vi "Connect.vi"(8 "error in":errorcluster, 11 "ThorlabsLabJack in":refnum<class "ThorlabsLabJack.lvclass">) -> (0 "error out":errorcluster, 3 "ThorlabsLabJack out":refnum<class "ThorlabsLabJack.lvclass">)   [LabVIEW 2018, in "ThorlabsLabJack.lvlib" / "ThorlabsLabJack.lvclass"]
uses:
  ThorlabsLabJack.lvclass
  ThorlabsLabJack.lvclass/ThorlabsLabJack.ctl
  C:/AME Test Engineering/LabVIEW/PPLs/Axis/Thorlabs/Thorlabs.MotionControl.IntegratedStepperMotorsCLI.dll
  PPLs/Axis/Thorlabs/Thorlabs.MotionControl.IntegratedStepperMotorsCLI.dll
  PPLs/Axis/Parent/Axis.lvlibp/Axis.lvclass
  C:/Projects/LWS_Base/trunk/LabVIEW/PPLs/Configuration/Axis.lvlibp/Axis.lvclass
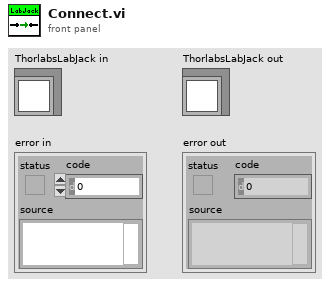
[diagram p1: front panel]
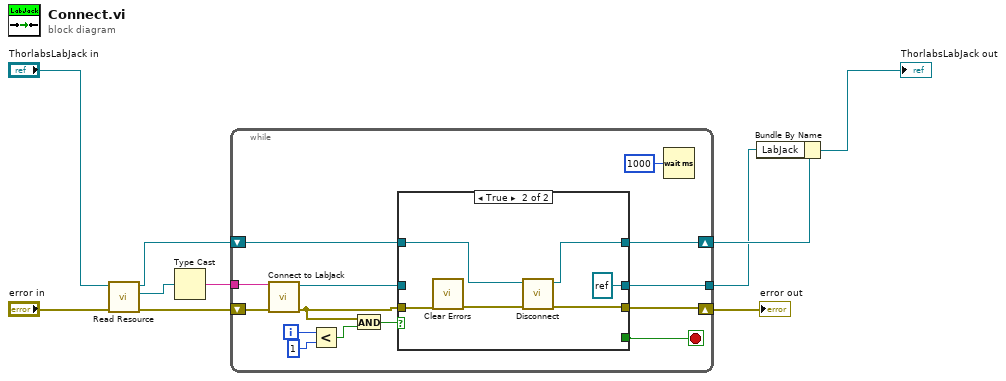
[diagram p0: block diagram]
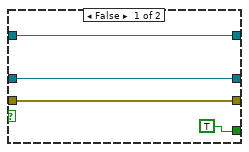
[diagram p2: hidden frame]
diagram:
  n1 = call "Read Resource.vi"("error in"="error in", "Axis in"="ThorlabsLabJack in") -> ("error out"=w6:errorcluster, "Resource"=w9:refnum<visa-resource-name>, "Axis out"=w8:refnum<class "ThorlabsLabJack.lvclass">)  [unwired: 7 in]
  n2 = Type Cast(x=w9) -> (*(type *) &x=w7:string)  [unwired: 1 in]
  n3 = while {
    shift-right: [w12] -> w5
    shift-left: w8 -> [w13]
    tunnel: w7 -> [w22]
    shift-right: [w15] -> w1
    shift-left: w6 -> [w23]
    tunnel: [w14] -> w2
    i -> [w20]
    stop <- w11 stop-if-true
    n4 = call "Connect to LabJack.vi"("Error In"=w23, "Serial Number"=w22) -> ("Error Out"=w17:errorcluster, "LabJack"=w16:refnum<k24>)  [unwired: 8 in]
    n5 = Less?(x=w20, y=1) -> (x < y?=w21:bool)
    n6 = And(x=w17, y=w21) -> (x .and. y?=w18:bool)
    n7 = case shown="True" w18 {
      tunnel: w17 -> [w27 w34]
      tunnel: w16 -> [w28 _]
      tunnel: [w28 refnum<k24> refnum ("LabJack")] -> w14
      tunnel: [w27 w32] -> w15
      tunnel: w13 -> [w26 w31]
      tunnel: [w26 w30] -> w12
      tunnel: [TRUE _] -> w11
      frame False {
      }
      frame True {
        n8 = call <vilib>:"Clear Errors.vi"("error in (no error)"=w34) -> ("error out"=w33:errorcluster)  [unwired: 5 in, 1 out]
        n9 = call-dynamic "Disconnect.vi"("error in"=w33, "ThorlabsLabJack in"=w31) -> ("error out"=w32:errorcluster, "ThorlabsLabJack out"=w30:refnum<class "ThorlabsLabJack.lvclass">)  [unwired: 8 in]
      }
    }
    n10 = Wait (ms)(milliseconds to wait=u32 1000) -> ()  [unwired: 1 out]
  }
  "error out" <- w1
  n11 = Bundle By Name(cluster=w5, "LabJack"=w2) -> (→"ThorlabsLabJack out":refnum<class "ThorlabsLabJack.lvclass">)
